vi "ErrorStructureDrawer.vi"(6 "Variant in":variant, 7 "Shift Pressed?":bool, 8 "error in (no error)":errorcluster, 10 "QD Combo Box Ref":refnum<vi>, 11 "QD Launch VI Ref":refnum<vi>) -> (0 "error out":errorcluster, 4 "Variant out":variant)   [LabVIEW 2017]
doc: "Implements the typical LabVIEW error handling:\n- Encloses code in a case structure\n- Wires an error control and indicator to that structure\n- Adds the control and indicator to the connetor pane.\n\nExisting error control and/or indicator are used if present, otherwise they are created.\n\nDefault Shortcut - [E]"
uses:
  ErrorStructureDrawer/ErrorStructureDrawer.lvlib
panel:
  in  "Undo Name":string="Create Inputs and/or Outputs"
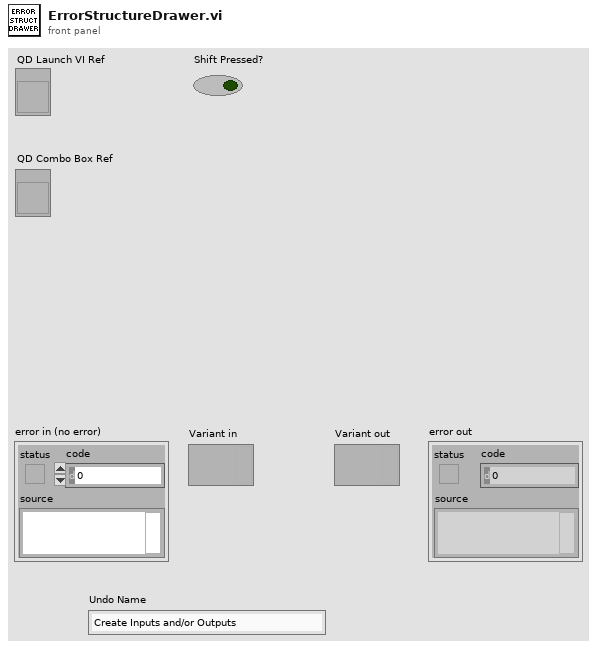
[diagram p1: front panel]
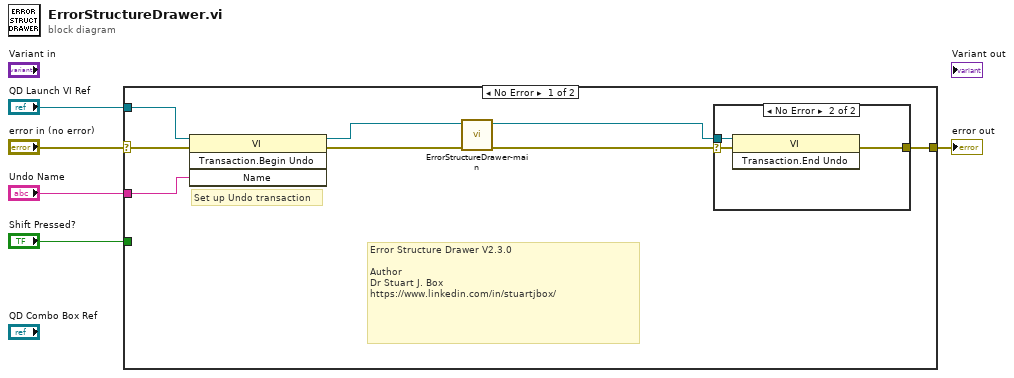
[diagram p0: block diagram]
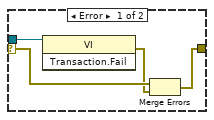
[diagram p2: hidden frame]
diagram:
  n1 = case shown="No Error" "error in (no error)" {
    selector: "error in (no error)" -> [w13 w21]
    tunnel: [w11 w21] -> w4
    tunnel: "Shift Pressed?" -> [_ _]
    tunnel: "QD Launch VI Ref" -> [w12 _]
    tunnel: "Undo Name" -> [w10 _]
    frame No Error {
      # "Error Structure Drawer V2.3.0\n\nAuthor\nDr Stuart J. Box\nhttps://www.linkedin.com/in/stuartjbox/"
      # "Set up Undo transaction"
      n2 = invoke class="VI" method="Transaction.Begin Undo"(reference=w12, error in=w13, "Name"=w10) -> (reference out=w8:refnum<vi>, error out=w9:errorcluster)  [unwired: 1 in, 2 out]
      n3 = call "ErrorStructureDrawer-main.vi"("Error In"=w9, "VI reference"=w8) -> ("Error Out"=w6:errorcluster, "VI reference (dup)"=w7:refnum<vi>)  [unwired: 8 in]
      n4 = case shown="No Error" w6 {
        selector: w6 -> [w16 w18]
        tunnel: w7 -> [w17 w19]
        tunnel: [w14 w20] -> w11
        frame Error {
          n5 = invoke class="VI" method="Transaction.Fail"(reference=w17) -> (error out=w15:errorcluster)  [unwired: 2 in, 2 out]
          n6 = Merge Errors(w16, w15) -> (w14:errorcluster)
        }
        frame No Error {
          n7 = invoke class="VI" method="Transaction.End Undo"(reference=w19, error in=w18) -> (error out=w20:errorcluster)  [unwired: 1 in, 2 out]
        }
      }
    }
    frame Error {
    }
  }
  "error out" <- w4
